vi "close_all.vi"(8 "error in (no error)":errorcluster, 11 "DDS Settings":T1={"Enable DDS"=TRUE, "Array of DDS Boxes"=[]} {"Array of DDS Boxes"."Array of DDS Channels (4)"."Channel Parameters"."Ref Clock Rate [MHz]" min=0.0}) -> (0 "error out":errorcluster)   [LabVIEW 2014, in "Experiment.lvclass"]
uses:
  Experiment.lvclass
  DDS/DDS_Settings_Cluster.ctl
  DDS/DDS Library/Controls/DDS Box Array.ctl
  DDS/DDS Library/Controls/DDS Box Cluster.ctl
  DDS/DDS Library/Controls/DDS Box Device Reference.ctl
  <vilib>/ni845x/ni845x.llb/ni845xControl.ctl
  DDS/DDS Library/Controls/DDS Channel Array.ctl
  DDS/DDS Library/Controls/DDS Channel.ctl
  DDS/DDS Library/Controls/DDS Channel Parameters.ctl
  DDS/DDS Library/Controls/DDS RAM Destination.ctl
  DDS/DDS Library/Controls/DDS Profile Array.ctl
  DDS/DDS Library/Controls/DDS Profile.ctl
  DDS/DDS Library/Controls/DDS RAM Mode.ctl
  DDS/DDS Library/Controls/DDS RAM Timestep.ctl
  DDS/DDS.lvclass
  DDS/DDS Library/DDS.lvlib
panel:
  # "f/f/A"
  # "Mag"
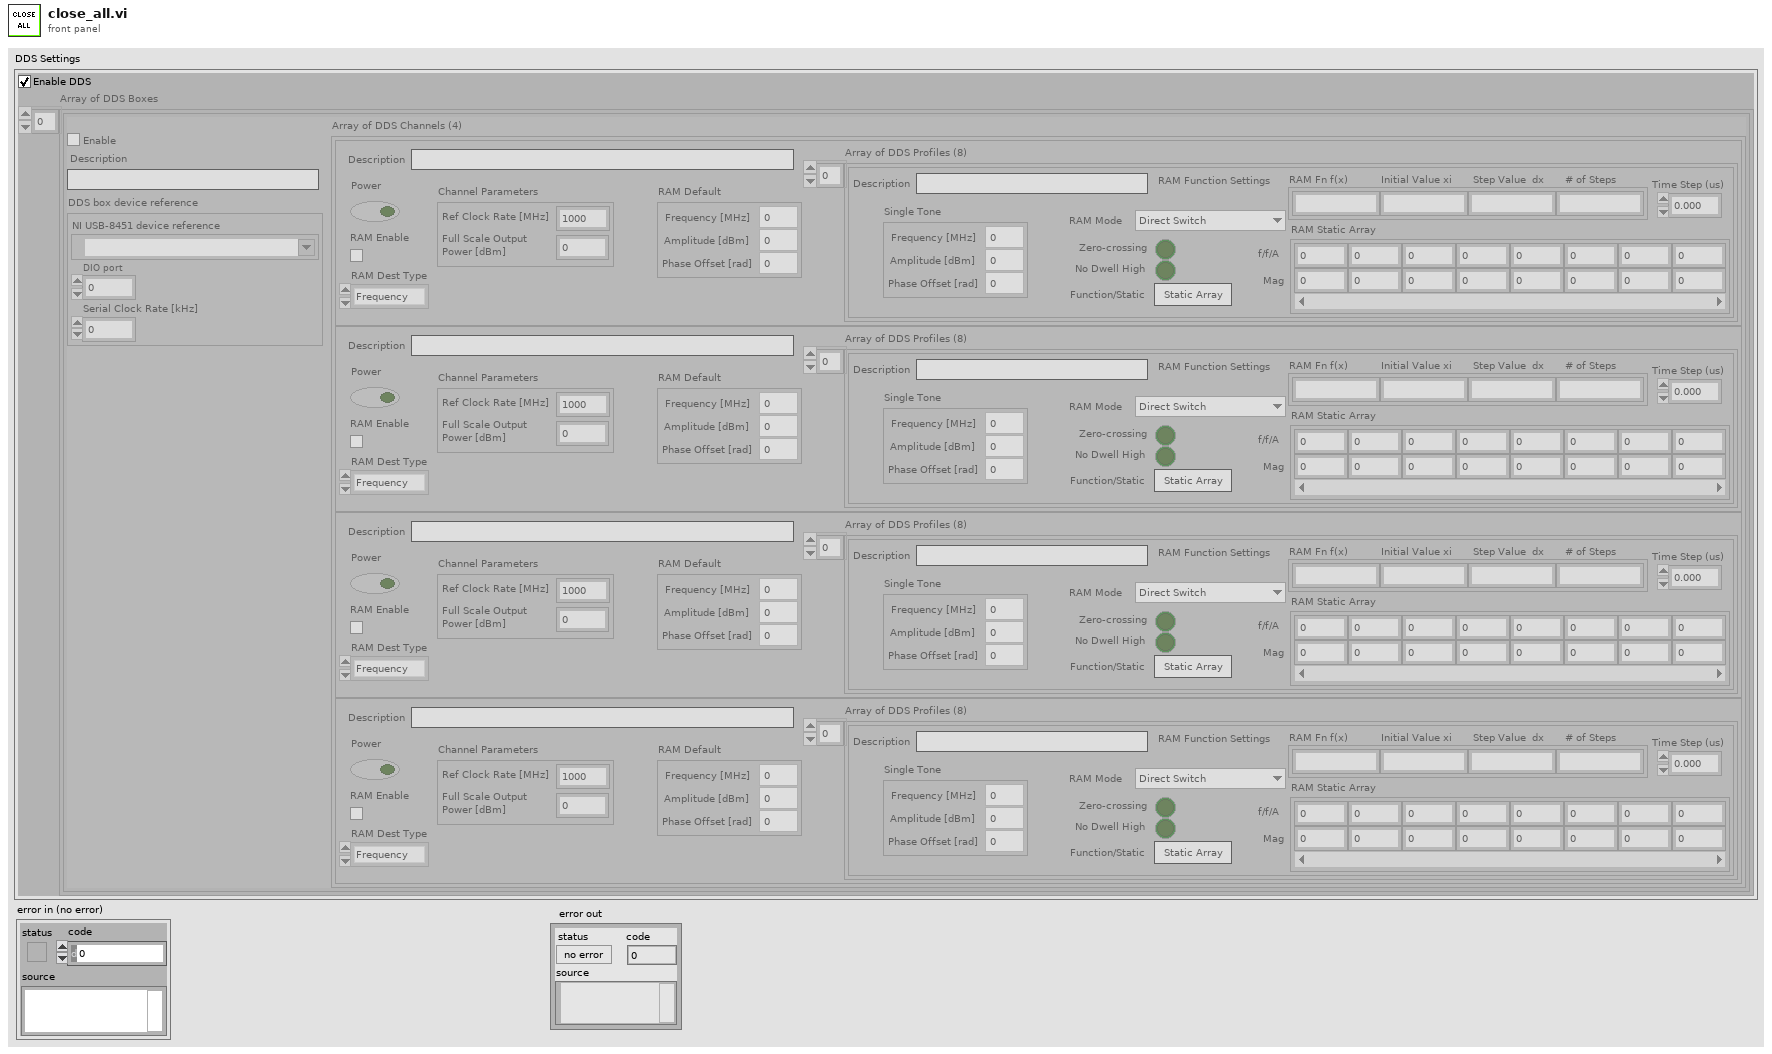
[diagram p1: front panel]
types:
  T1 = typedef "DDS.lvclass/DDS_Settings_Cluster.ctl" = cluster{"Enable DDS":bool, "Array of DDS Boxes":T2}
  T2 = typedef "DDS.lvlib/DDS Box Array.ctl" = T3[]
  T3 = typedef "DDS.lvlib/DDS Box Cluster.ctl" = cluster{"DDS box device reference":T4, "Array of DDS Channels (4)":T6, "Enable":bool, "Description":string}
  T4 = typedef "DDS.lvlib/DDS Box Device Reference.ctl" = cluster{"NI USB-8451 device reference":T5, "DIO port":u8, "Serial Clock Rate [kHz]":u16}
  T5 = typedef "ni845xControl.ctl" = refnum<k21>
  T6 = typedef "DDS.lvlib/DDS Channel Array.ctl" = T7[]
  T7 = typedef "DDS.lvlib/DDS Channel.ctl" = cluster{"Power":bool, "Channel Parameters":T8, "RAM Enable":bool, "RAM Dest Type":T9, "RAM Default":cluster{"Frequency [MHz]":dbl, "Amplitude [dBm]":dbl, "Phase Offset [rad]":dbl}, "Array of DDS Profiles (8)":T10, "Description":string}
  T8 = typedef "DDS.lvlib/DDS Channel Parameters.ctl" = cluster{"Ref Clock Rate [MHz]":dbl, "Full Scale Output\nPower [dBm]":dbl}
  T9 = typedef "DDS.lvlib/DDS RAM Destination.ctl" = enum16{"Frequency", "Phase", "Amplitude", "Polar"}
  T10 = typedef "DDS.lvlib/DDS Profile Array.ctl" = T11[]
  T11 = typedef "DDS.lvlib/DDS Profile.ctl" = cluster{"Single Tone":cluster{"Frequency [MHz]":dbl, "Amplitude [dBm]":dbl, "Phase Offset [rad]":dbl}, "RAM Mode ":T12, "Zero-crossing":bool, "No Dwell High":bool, "Function/Static":bool, "RAM Function Settings":string[], "RAM Static Array":dbl[][], "Description":string, "Time Step (us)":T13}
  T12 = typedef "DDS.lvlib/DDS RAM mode.ctl" = enum16{"Direct Switch", "Ramp Up", "Bidirectional Ramp", "Continuous Bidirectional Ramp", "Continuous Recirculate", "Direct Switch 2", "Direct Switch 3", "Direct Switch 4"}
  T13 = typedef "DDS.lvlib/DDS RAM Timestep.ctl" = dbl
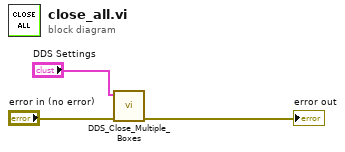
[diagram p0: block diagram]
diagram:
  n1 = call "DDS_Close_Multiple_Boxes.vi"("error in (no error)"="error in (no error)", "DDS Settings"="DDS Settings") -> ("error out"=→"error out":errorcluster)  [unwired: 9 in]
